vi "Get Env data (oneshot) (D).vi"(0 "VISA resource name in":refnum<visa-resource-name>, 3 "Error In":errorcluster) -> (7 "VISA resource name out":refnum<visa-resource-name>, 8 "STATE_Buffer":string, 9 "ACK":bool, 10 "Error out":errorcluster)   [LabVIEW 2015]
uses:
  Ctls/Cmd str.ctl
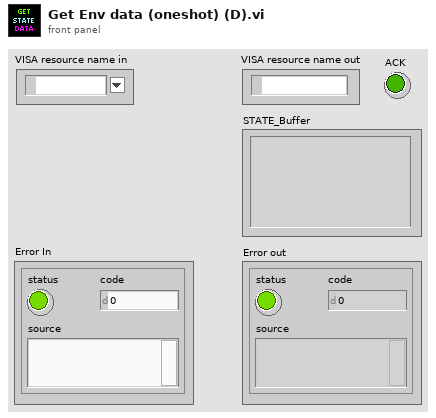
[diagram p1: front panel]
types:
  T1 = typedef "Cmd str.ctl" = string
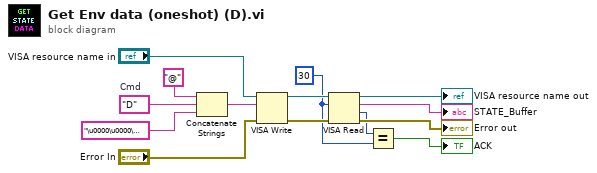
[diagram p0: block diagram]
diagram:
  w1 = u32 30 ("byte count")
  w10 = T1 "D"  # Cmd
  n1 = Concatenate Strings("@" ("string"), w10, "\u0000\u0000\u0000\u0000" ("4 byte config str")) -> (w11:string)
  n2 = VISA Write(VISA resource name="VISA resource name in", write buffer=w11, error in (no error)="Error In") -> (VISA resource name out=w13:refnum<visa-resource-name>, error out=w12:errorcluster)  [unwired: 1 out]
  n3 = VISA Read(VISA resource name=w13, byte count=w1, error in (no error)=w12) -> (VISA resource name out=→"VISA resource name out":refnum<visa-resource-name>, read buffer=→"STATE_Buffer":string, return count=w2:u32, error out=→"Error out":errorcluster)
  n4 = Equal?(x=w2, y=w1) -> (x = y?=→"ACK":bool)
